vi "Select averaging.vi"(8 "error in (no error)":errorcluster, 10 "Averaging":T1, 11 "VISA resource name":refnum<visa-resource-name>="GPIB0::21::INSTR") -> (0 "error out":errorcluster, 3 "VISA resource name out":refnum<visa-resource-name>)   [LabVIEW 2017]
uses:
  Averaging control.ctl
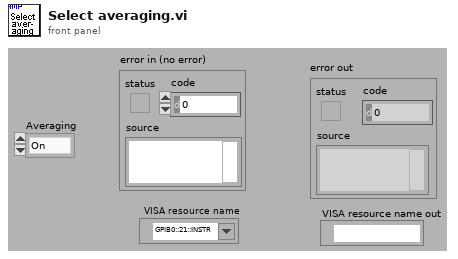
[diagram p1: front panel]
types:
  T1 = typedef "Averaging control.ctl" = enum16{"On", "Off"}
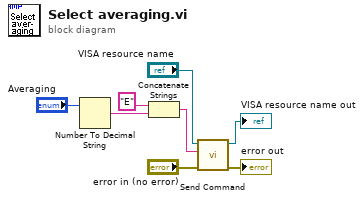
[diagram p0: block diagram]
diagram:
  n1 = Number To Decimal String(number="Averaging") -> (decimal integer string=w2:string)  [unwired: 1 in]
  n2 = Concatenate Strings("E" ("string"), w2) -> (w1:string)
  n3 = call "Send Command.vi"("error in (no error)"="error in (no error)", "write buffer"=w1, "VISA resource name"="VISA resource name") -> ("error out"=→"error out":errorcluster, "VISA resource name out"=→"VISA resource name out":refnum<visa-resource-name>)  [unwired: 7 in]
